vi "waitForNewImage.vi"(8 "error in (no error)":errorcluster, 9 "timeout_s":dbl=nan, 10 "delay":bool=TRUE, 11 "Camera in":refnum<class "Camera.lvclass">) -> (0 "error out":errorcluster, 3 "Camera out":refnum<class "Camera.lvclass">)   [LabVIEW 2020, in "Camera.lvclass"]
doc: "Waits for the first available image in the recorder memory. In recorder mode 'sequence non\nblocking', 'ring buffer'. and 'fifo', the function record.vi returns immediately.\nTherefore, this function can be used to wait for images from the camera before calling\nimage.vi, images.vi, or image_average.vi."
uses:
  Camera.lvclass
  Camera.lvclass/Camera.ctl
  Recorder.lvlib
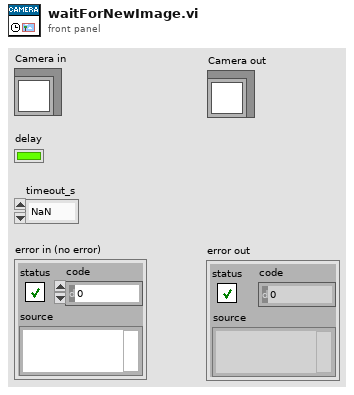
[diagram p1: front panel]
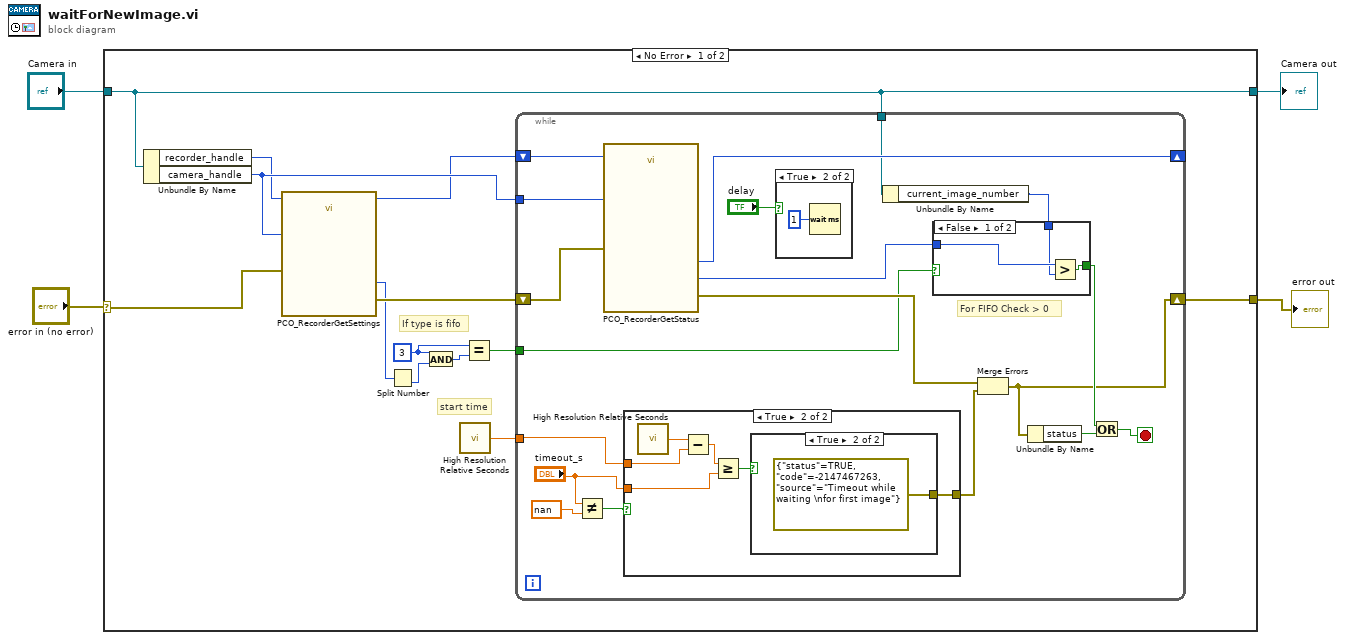
[diagram p0: block diagram]
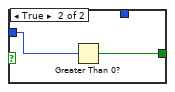
[diagram p2: hidden frame]
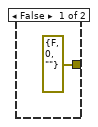
[diagram p3: hidden frame]
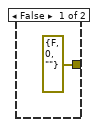
[diagram p4: hidden frame]
diagram:
  n1 = case shown="No Error" "error in (no error)" {
    selector: "error in (no error)" -> [w13 w53]
    tunnel: [w5 w53] -> w2
    tunnel: [w16 w52] -> w1
    tunnel: "Camera in" -> [w16 w52]
    frame No Error {
      w7 = u16 3 ("dwRecMode")
      # "If type is fifo"
      # "start time"
      n2 = Unbundle By Name(w16) -> ("recorder_handle"=w14:u64, "camera_handle"=w15:u64)
      n3 = call "PCO_RecorderGetSettings.vi"("phRec"=w14, "phCam"=w15, "error in (no error)"=w13) -> ("phRec out"=w11:u64, "dwRecMode"=w10:u32, "error out"=w12:errorcluster)  [unwired: 4 in, 6 out]
      n4 = Split Number(x=w10) -> (lo(x)=w9:u16)  [unwired: 1 out]
      n5 = And(x=w7, y=w9) -> (x .and. y?=w8:u16)
      n6 = call "High Resolution Relative Seconds.vi"() -> ("relative seconds"=w17:dbl)
      n7 = Equal?(x=w7, y=w8) -> (x = y?=w6:bool)
      n8 = while {
        shift-right: [w24] -> w5
        shift-left: w12 -> [w35]
        shift-right: [w34] -> _
        shift-left: w11 -> [w36]
        tunnel: w15 -> [w33]
        tunnel: w17 -> [w27]
        tunnel: w16 -> [w20]
        tunnel: w6 -> [w18]
        stop <- w30 stop-if-true
        # "For FIFO Check > 0"
        n9 = Not Equal?(x="timeout_s", y=nan) -> (x != y?=w28:bool)
        n10 = call "PCO_RecorderGetStatus.vi"("phRec"=w36, "phCam"=w33, "error in (no error)"=w35) -> ("dwProcImgCount"=w21:u32, "phRec out"=w34:u64, "error out"=w25:errorcluster)  [unwired: 5 in, 9 out]
        n11 = case shown="True" w28 {
          tunnel: w27 -> [_ w47]
          tunnel: "timeout_s" -> [_ w45]
          tunnel: [errorcluster {"status"=FALSE, "code"=0, "source"=""} ("error constant") w43] -> w26
          frame False {
          }
          frame True {
            n12 = call "High Resolution Relative Seconds.vi"() -> ("relative seconds"=w48:dbl)
            n13 = Subtract(x=w48, y=w47) -> (x-y=w46:dbl)
            n14 = Greater Or Equal?(x=w46, y=w45) -> (x >= y?=w44:bool)
            n15 = case shown="True" w44 {
              tunnel: [errorcluster {"status"=FALSE, "code"=0, "source"=""} ("error constant") errorcluster {"status"=TRUE, "code"=-2147467263, "source"="Timeout while waiting \nfor first image"} ("error constant")] -> w43
              frame False {
              }
              frame True {
              }
            }
          }
        }
        n16 = case shown="True" "delay" {
          frame False {
          }
          frame True {
            n17 = Wait (ms)(milliseconds to wait=u32 1) -> ()  [unwired: 1 out]
          }
        }
        n18 = Unbundle By Name(w20) -> ("current_image_number"=w19:u32)
        n19 = case shown="False" w18 {
          tunnel: [w39 w40] -> w31
          tunnel: w21 -> [w38 w41]
          tunnel: w19 -> [w37 _]
          frame False {
            n20 = Greater?(x=w38, y=w37) -> (0:w39:bool)
          }
          frame True {
            n21 = Greater Than 0?(x=w41) -> (x > 0?=w40:bool)
          }
        }
        n22 = Merge Errors(w25, w26) -> (w24:errorcluster)
        n23 = Unbundle By Name(w24) -> ("status"=w32:bool)
        n24 = Or(x=w31, y=w32) -> (x .or. y?=w30:bool)
      }
    }
    frame Error {
    }
  }
  "error out" <- w2
  "Camera out" <- w1
